vi "General-GenerateSineWaveForm.vi"(0 "tiempo (s)":sgl, 1 "#samples":u32, 2 "Amplitud":dbl, 3 "frecuencia":dbl, 4 "Fs (S/s)":dbl, 5 "df":dbl[](array[numeric])) -> (7 "Waveform":waveform(dbl)(graph))   [LabVIEW 2010]
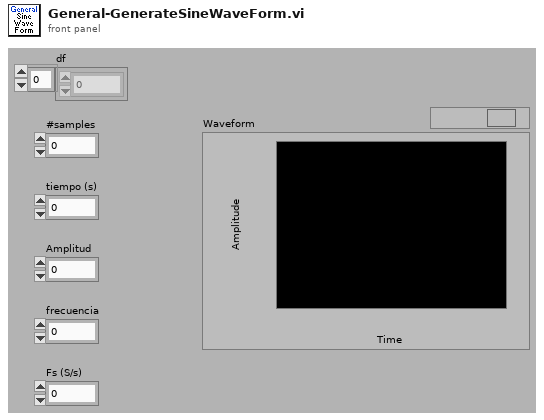
[diagram p1: front panel]
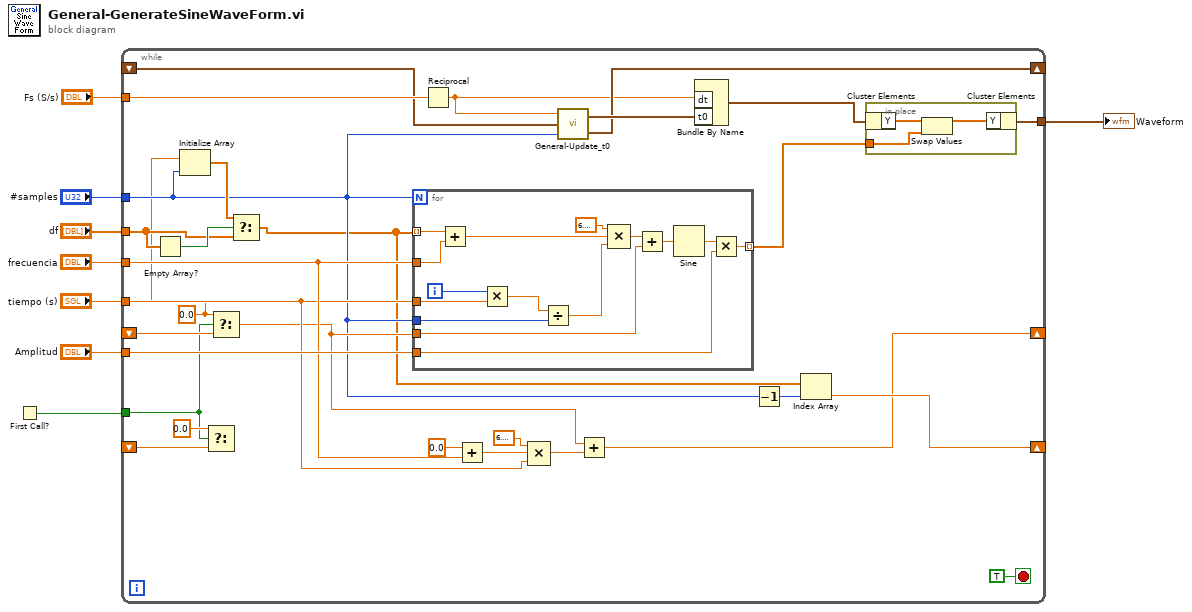
[diagram p0: block diagram]
diagram:
  n1 = First Call?() -> (First Call?: T/F=w1:bool)
  n2 = while {
    tunnel: "#samples" -> [w11]
    tunnel: "tiempo (s)" -> [w26]
    tunnel: "frecuencia" -> [w29]
    tunnel: "Amplitud" -> [w37]
    shift-right: [w24] -> _
    shift-left: _ -> [w21]
    tunnel: "Fs (S/s)" -> [w36]
    shift-right: [w32] -> _
    shift-left: _ -> [w34]
    tunnel: [w22] -> w8
    tunnel: "df" -> [w13]
    shift-right: [w30] -> _
    shift-left: _ -> [w18]
    tunnel: w1 -> [w17]
    stop <- TRUE stop-if-true
    w10 = 0.0 ("t")
    n3 = Empty Array?(array=w13) -> (empty?=w14:bool)
    n4 = Initialize Array(w10, w11) -> (w12:dbl[])
    n5 = Select(t=0.0, s=w17, f=w18) -> ()  [unwired: 1 out]
    n6 = Select(t=w10, s=w17, f=w21) -> (s? t:f=w20:dbl)
    n7 = Select(t=w12, s=w14, f=w13) -> (s? t:f=w9:dbl[])
    n8 = for {
      N: w11 -> [_]
      tunnel: w26 -> [w55]
      tunnel: w29 -> [w46]
      tunnel: w20 -> [w52]
      tunnel: w37 -> [w50]
      tunnel: w11 -> [w44]
      tunnel: w9 -> [w43] mode=indexing
      tunnel: [w42] -> w15 mode=indexing
      i -> [w56]
      n9 = Add(x=w43, y=w46) -> (x+y=w45:dbl)
      n10 = Multiply(x=w56, y=w55) -> (x*y=w54:sgl)
      n11 = Divide(x=w54, y=w44) -> (x/y=w48:sgl)
      n12 = Compound Arithmetic op=MULTIPLY(6.283185307179586, w45, w48) -> (w47:dbl)
      n13 = Add(x=w47, y=w52) -> (x+y=w53:dbl)
      n14 = Sine(x=w53) -> (sin(x)=w51:dbl)
      n15 = Multiply(x=w51, y=w50) -> (x*y=w42:dbl)
    }
    n16 = Reciprocal(x=w36) -> (1/x=w23:dbl)
    n17 = Add(x=0.0, y=w29) -> (x+y=w27:dbl)
    n18 = Compound Arithmetic op=MULTIPLY(6.283185307179586, w27, w26) -> (w25:dbl)
    n19 = call "General-Update_t0.vi"("#samples"=w11, "t0 IN"=w34, "dt"=w23) -> ("tf new"=w32:timestamp, "t0 OUT"=w33:timestamp)
    n20 = Add(x=w20, y=w25) -> (x+y=w24:dbl)
    n21 = Bundle By Name("dt"=w23, "t0"=w33) -> (w35:waveform(dbl))  [unwired: 1 in]
    n22 = Decrement(x=w11) -> (x-1=w31:u32)
    n23 = Index Array(array=w9, index=w31) -> (element=w30:dbl)
    n24 = in-place {
      in-place-border: w15 -> [w39]
      n25 = in-place-cluster #1(w35) -> ("Y"=w41:dbl[])
      n26 = Swap Values(12:w41, 14:w39) -> (1:w40:dbl[])  [unwired: 1 in, 1 out]
      n27 = in-place-cluster #1("Y"=w40) -> (w22:waveform(dbl))
    }
  }
  "Waveform" <- w8
